vi "Perform Action.vi"(8 "error in":errorcluster, 10 "Input":variant, 11 "Thermometer DAQmx RTD Cont CFG in":refnum<class "Thermometer DAQmx RTD Cont CFG.lvclass">) -> (0 "error out":errorcluster, 2 "Output":variant, 3 "Thermometer DAQmx RTD Cont CFG out":refnum<class "Thermometer DAQmx RTD Cont CFG.lvclass">)   [LabVIEW 2023, in "Thermometer DAQmx RTD Cont CFG.lvclass"]
uses:
  Thermometer DAQmx RTD Cont CFG.lvclass
  DAQmx/DAQmx Base CFG/DAQmx Base CFG.lvclass/DAQmx Base CFG.ctl
  <vilib>/DAQmx/read.llb/DAQmx Read (Analog 2D DBL NChan NSamp).vi
  <vilib>/DAQmx/miscellaneous.llb/DAQmx Fill In Error Info.vi
  DAQmx/DAQmx Base CFG/DAQmx Base CFG.lvclass
  <resource>/objmgr/daqmx.rc
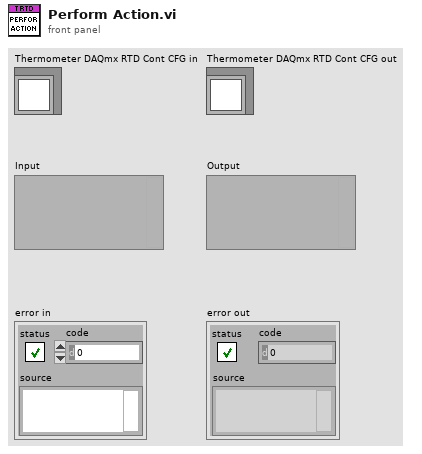
[diagram p1: front panel]
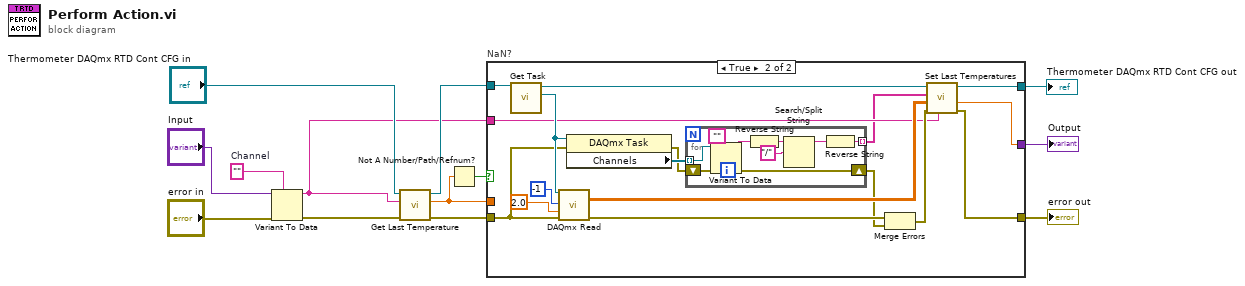
[diagram p0: block diagram]
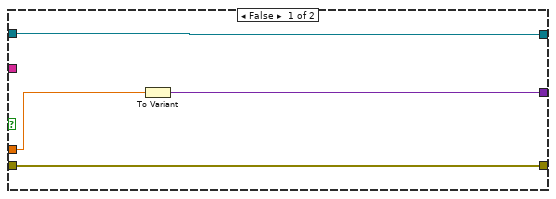
[diagram p2: hidden frame]
diagram:
  w1 = ""  # Channel
  n1 = Variant To Data(error in="error in", type=w1, Variant="Input") -> (data=w2:string, error out=w12:errorcluster)
  n2 = call "Get Last Temperature.vi"("error in"=w12, "Channel"=w2, "Thermometer DAQmx RTD Cont CFG in"="Thermometer DAQmx RTD Cont CFG in") -> ("error out"=w7:errorcluster, "Temperature"=w5:dbl, "Thermometer DAQmx RTD Cont CFG out"=w8:refnum<class "Thermometer DAQmx RTD Cont CFG.lvclass">)  [unwired: 6 in]
  n3 = Not A Number/Path/Refnum?(number/path/refnum=w5) -> (NaN/Path/Refnum?=w9:bool)
  n4 = case "NaN?" shown="True" w9 {
    tunnel: w8 -> [w15 w34]
    tunnel: w7 -> [w14 w26]
    tunnel: [w14 w30] -> w6
    tunnel: [w16 w22] -> w4
    tunnel: [w15 w28] -> w3
    tunnel: w5 -> [w17 _]
    tunnel: w2 -> [_ w23]
    frame False {
      n5 = To Variant(anything=w17) -> (Variant=w16:variant)
    }
    frame True {
      n6 = call "Get Task.vi"("DAQmx Base CFG in"=w34) -> ("Task"=w27:refnum<k21>, "DAQmx Base CFG out"=w29:refnum<class "Thermometer DAQmx RTD Cont CFG.lvclass">)  [unwired: 9 in]
      n7 = call-poly <vilib>:"DAQmx Read.vi"("task/channels in"=w27, "number of samples per channel"=-1, "timeout"=2.0, "error in"=w26) -> ("data"=w24:dbl[][], "error out"=w31:errorcluster)  [unwired: 9 in, 1 out]
      n8 = property class="DAQmx Task"(reference=w27, error in=w26) -> (error out=w20:errorcluster, "Channels"=w21:refnum<k21>[])  [unwired: 1 out]
      n9 = for {
        tunnel: w21 -> [w43] mode=indexing
        shift-right: [w38] -> w19
        shift-left: w20 -> [w42]
        tunnel: [w35] -> w18 mode=indexing
        n10 = Variant To Data(error in=w42, type="", Variant=w43) -> (data=w40:string, error out=w38:errorcluster)
        n11 = Reverse String(1:w40) -> (0:w37:string)
        n12 = Search/Split String(string=w37, search string/char (-)="/") -> (substring before match=w36:string)  [unwired: 1 in, 2 out]
        n13 = Reverse String(1:w36) -> (0:w35:string)
      }
      n14 = Merge Errors(w31, w19) -> (w25:errorcluster)
      n15 = call "Set Last Temperatures.vi"("Read Channel Ident"=w23, "error in"=w25, "Temperatures"=w24, "Channel Idents"=w18, "Thermometer DAQmx RTD Cont CFG in"=w29) -> ("error out"=w30:errorcluster, "Temperature"=w22:dbl, "Thermometer DAQmx RTD Cont CFG out"=w28:refnum<class "Thermometer DAQmx RTD Cont CFG.lvclass">)  [unwired: 4 in]
    }
  }
  "error out" <- w6
  "Thermometer DAQmx RTD Cont CFG out" <- w3
  "Output" <- w4
